vi "LADS-Console-LV-TCP.vi"() -> ()   [LabVIEW 2023]
doc: "Demonstrates how to open a connection to an TCP server, read the data being sent, and display the data on a chart. This VI is designed to stop if the TCP connection is terminated."
panel:
  in  "OK Button":bool
  out "Numeric":dbl
  out "Waveform Chart":dbl[](graph)
  out "Connection 2":string
  in  "Server Closed 2":string="The server VI closed the connection."
  out "?":string
  out "?":string
  out "Connection 1":string
  in  "Server Closed":string="The server VI closed the connection."
  # "Overview: Demonstrates the use of the TCP functions to connect to a TCP server VI and receive data.\nInstructions:\n1. Ensure Simple TCP - Server.vi is already running.\n2. Run the VI.\n3. Click Stop to stop the VI. Note that if you stop the server VI, this VI will stop automatically."
  # "TS\n\nA0"
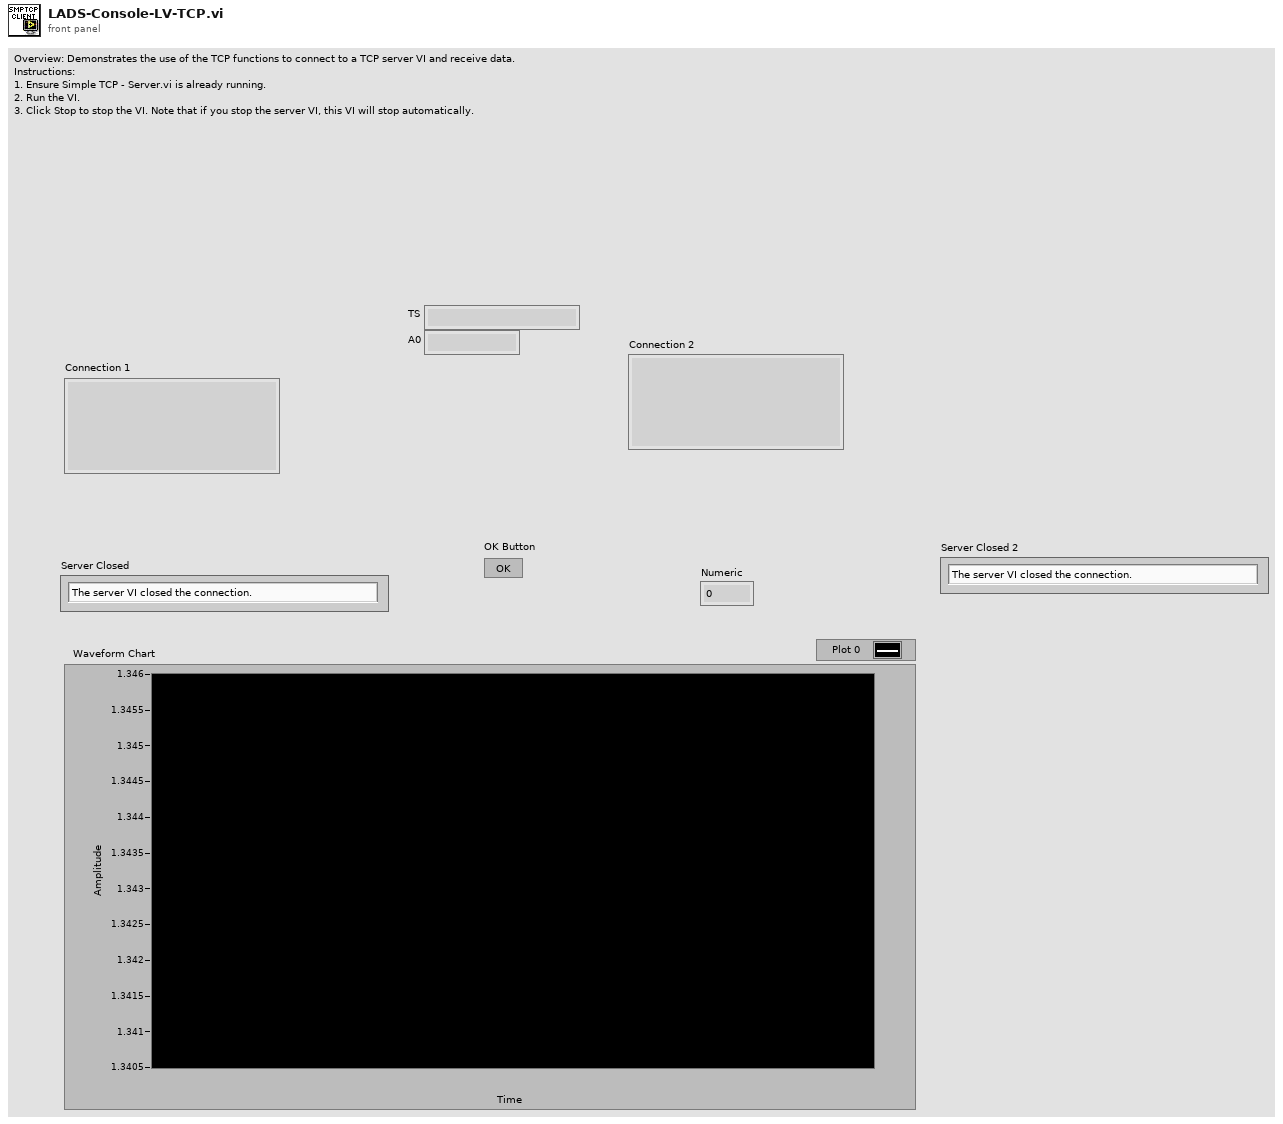
[diagram p1: front panel]
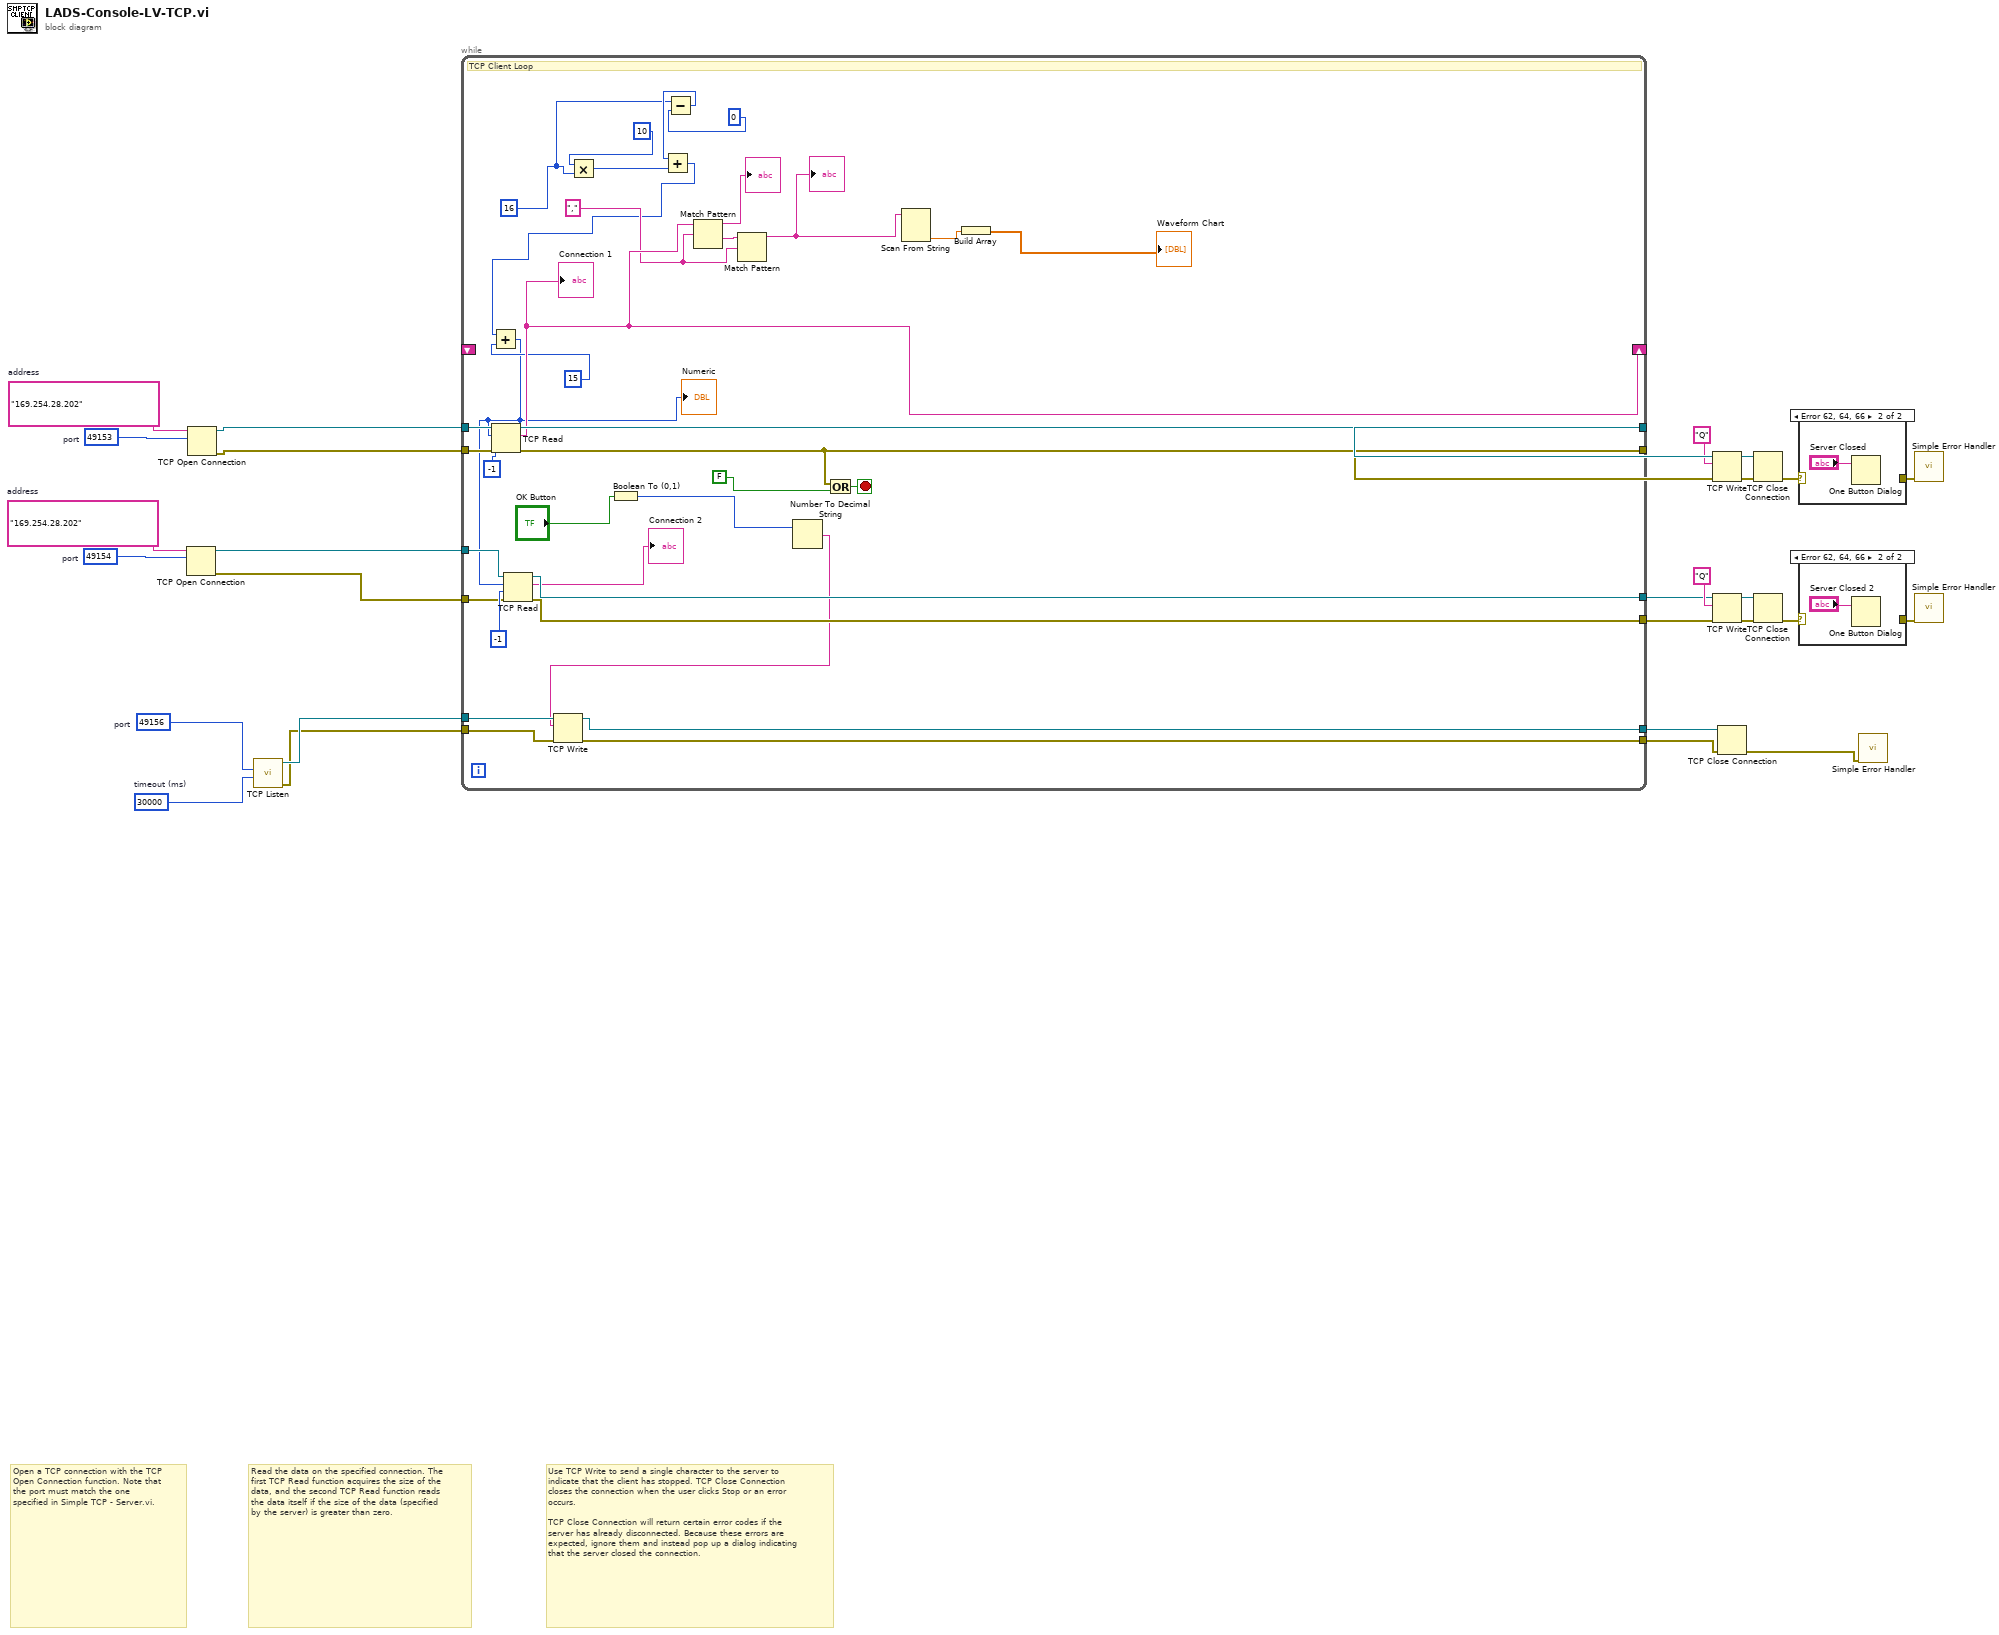
[diagram p0: block diagram]
diagram:
  w4 = 30000  # timeout (ms)
  w3 = u16 49156  # port
  w17 = u16 49154  # port
  w18 = "169.254.28.202"  # address
  w19 = u16 49153  # port
  w20 = "169.254.28.202"  # address
  # "Use TCP Write to send a single character to the server to indicate that the client has stopped. TCP Close Connection closes the connection when the user clicks Stop or an error occurs.\n\nTCP Close Connection will return certain error codes if the server has already disconnected. Because these errors are expected, ignore them and instead pop up a dialog indicating that the server closed the connection."
  # "Read the data on the specified connection. The first TCP Read function acquires the size of the data, and the second TCP Read function reads the data itself if the size of the data (specified by the server) is greater than zero."
  # "Open a TCP connection with the TCP Open Connection function. Note that the port must match the one specified in Simple TCP - Server.vi."
  n1 = TCP Open Connection(address=w18, remote port or service name=w17) -> (connection ID=w15:refnum<k5>, error out=w16:errorcluster)  [unwired: 3 in]
  n2 = TCP Open Connection(address=w20, remote port or service name=w19) -> (connection ID=w29:refnum<k5>, error out=w28:errorcluster)  [unwired: 3 in]
  n3 = call <vilib>:"TCP Listen.vi"("timeout ms (wait forever: -1)"=w4, "port"=w3) -> ("error out"=w1:errorcluster, "connection ID"=w2:refnum<k5>)  [unwired: 5 in, 3 out]
  n4 = while {
    tunnel: w28 -> [w63]
    tunnel: w29 -> [w64]
    tunnel: [w60] -> w26
    tunnel: [w59] -> w24
    shift-right: [w58] -> _
    shift-left: _ -> [_]
    tunnel: w16 -> [w52]
    tunnel: w15 -> [w51]
    tunnel: [w50] -> w9
    tunnel: [w49] -> w8
    tunnel: w2 -> [w37]
    tunnel: w1 -> [w36]
    tunnel: [w35] -> w6
    tunnel: [w34] -> w5
    stop <- w62 stop-if-true
    w33 = 16
    w54 = ","
    # "TCP Client Loop"
    n5 = Multiply(x=10, y=w33) -> (x*y=w47:i32)
    n6 = Boolean To (0,1)(Boolean="OK Button") -> (0, 1=w31:i16)
    n7 = Subtract(x=w33, y=0) -> (x-y=w45:i32)
    n8 = Add(x=w45, y=w47) -> (x+y=w44:i32)
    n9 = Add(x=w44, y=15) -> (x+y=w38:i32)
    "Numeric" <- w38
    n10 = TCP Read(connection ID=w64, bytes to read=w38, error in (no error)=w63, 9:-1 ("timeout ms (25000)")) -> (connection ID out=w60:refnum<k5>, data out=w58:string, error out=w59:errorcluster)  [unwired: 1 in]
    "Connection 1" <- w58
    n11 = TCP Read(connection ID=w51, bytes to read=w38, error in (no error)=w52, 9:-1 ("timeout ms (25000)")) -> (connection ID out=w50:refnum<k5>, data out=→"Connection 2":string, error out=w49:errorcluster)  [unwired: 1 in]
    n12 = Match Pattern(string=w58, regular expression=w54) -> (before substring=→"?":string, after substring=w56:string)  [unwired: 1 in, 2 out]
    n13 = Match Pattern(string=w56, regular expression=w54) -> (before substring=w42:string)  [unwired: 1 in, 3 out]
    "?" <- w42
    n14 = Number To Decimal String(number=w31) -> (decimal integer string=w30:string)  [unwired: 1 in]
    n15 = TCP Write(connection ID=w37, data in=w30, error in (no error)=w36) -> (connection ID out=w34:refnum<k5>, error out=w35:errorcluster)  [unwired: 1 in, 1 out]
    n16 = Or(x=w59, y=FALSE) -> (x .or. y?=w62:bool)
    n17 = Scan From String(input string=w42) -> (output 1=w40:dbl)  [unwired: 4 in, 3 out]
    n18 = Build Array(w40) -> (→"Waveform Chart":dbl[])
  }
  n19 = TCP Write(connection ID=w26, data in="Q", error in (no error)=w24) -> (connection ID out=w27:refnum<k5>, error out=w25:errorcluster)  [unwired: 2 out]
  n20 = TCP Write(connection ID=w9, data in="Q", error in (no error)=w8) -> (connection ID out=w14:refnum<k5>, error out=w13:errorcluster)  [unwired: 2 out]
  n21 = TCP Close Connection(connection ID=w5, error in (no error)=w6) -> (error out=w7:errorcluster)  [unwired: 1 in, 1 out]
  n22 = TCP Close Connection(connection ID=w27, error in (no error)=w25) -> (error out=w22:errorcluster)  [unwired: 1 in, 1 out]
  n23 = TCP Close Connection(connection ID=w14, error in (no error)=w13) -> (error out=w11:errorcluster)  [unwired: 1 in, 1 out]
  n24 = case shown="Error 62, 64, 66" w22 {
    selector: w22 -> [w65 _]
    tunnel: [w65 _] -> w21
    frame #0 {
    }
    frame #1 {
      n25 = One Button Dialog(message="Server Closed") -> ()  [unwired: 1 in, 1 out]
    }
  }
  n26 = case shown="Error 62, 64, 66" w11 {
    selector: w11 -> [w67 _]
    tunnel: [w67 _] -> w10
    frame #0 {
    }
    frame #1 {
      n27 = One Button Dialog(message="Server Closed 2") -> ()  [unwired: 1 in, 1 out]
    }
  }
  n28 = call <vilib>:"Simple Error Handler.vi"("error in (no error)"=w7) -> ()  [unwired: 4 in, 5 out]
  n29 = call <vilib>:"Simple Error Handler.vi"("error in (no error)"=w21) -> ()  [unwired: 4 in, 5 out]
  n30 = call <vilib>:"Simple Error Handler.vi"("error in (no error)"=w10) -> ()  [unwired: 4 in, 5 out]
